vi "02señalizacion 492.vi"(5 "Digitales":T1, 6 "Analogicas":dbl[](array[numeric]), 7 "Config Equipo":T3={"Modelo"="", "IP"="", "Puerto"=0, "Time Out"=0, "Med Princ"=0, "Time sin rx"=60, "Reintento"=60, "Ref PD 2"=200} {"Ref PD 2" max=10000 step=1; "Med Princ" items=["1", "2", "3", "4", "5", "6", "7", "8", "9", "10", "11", "12", "13", "14", "15", "16", "17", "18", "19", "20", "21", "22", "23", "24", "25", "26", "27", "28", "29", "30", "31", "32"]}) -> (2 "Error Logico":bool, 3 "Señalizacion":T2)   [LabVIEW 2010]
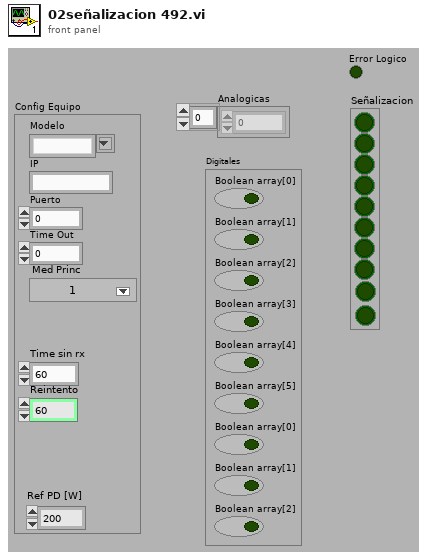
[diagram p1: front panel]
types:
  T1 = cluster{"Boolean array[0]":bool, "Boolean array[1]":bool, "Boolean array[2]":bool, "Boolean array[3]":bool, "Boolean array[4]":bool, "Boolean array[5]":bool, "Boolean array[0]":bool, "Boolean array[1]":bool, "Boolean array[2]":bool}
  T2 = cluster{bool, bool, bool, bool, bool, bool, bool, bool, bool, bool}
  T3 = cluster{"Modelo":string, "IP":string, "Puerto":u16, "Time Out":u16, "Med Princ":u16, "Time sin rx":u16, "Reintento":u16, "Ref PD 2":u16}
  T4 = cluster{bool, bool, bool, bool, bool, bool, bool, bool, bool, "Boolean array[5]":bool}
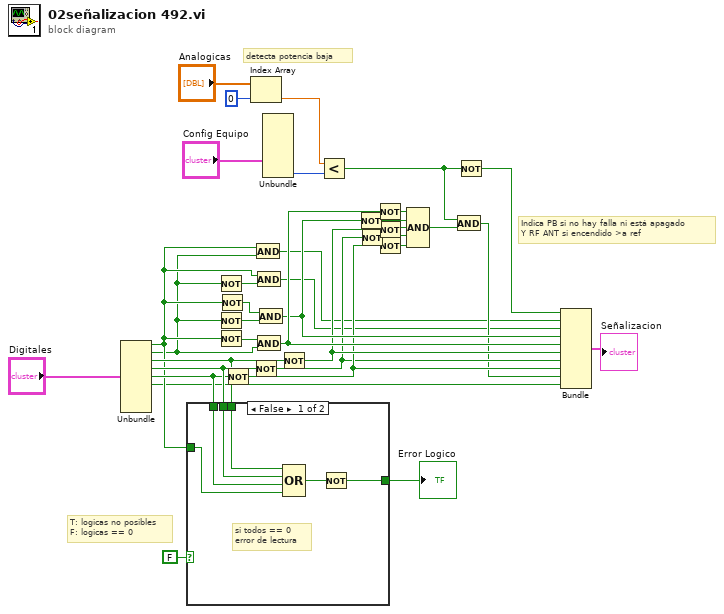
[diagram p0: block diagram]
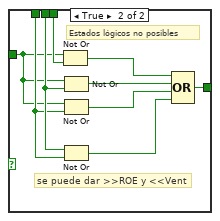
[diagram p2: hidden frame]
diagram:
  # "T: logicas no posibles\nF: logicas == 0"
  # "Indica PB si no hay falla ni está apagado\nY RF ANT si encendido >a ref"
  # "detecta potencia baja"
  n1 = Unbundle("Digitales") -> ("Boolean array[0]"=w29:bool, "Boolean array[1]"=w9:bool, "Boolean array[2]"=w31:bool, "Boolean array[3]"=w32:bool, "Boolean array[4]"=w30:bool, "Boolean array[5]"=w8:bool)  [unwired: 3 out]
  n2 = case shown="False" FALSE {
    tunnel: w32 -> [w40 w47]
    tunnel: w31 -> [w41 w46]
    tunnel: w30 -> [w39 w45]
    tunnel: w29 -> [w38 w44]
    tunnel: [w36 w43] -> w28
    frame False {
      # "si todos == 0\nerror de lectura"
      n3 = Compound Arithmetic op=OR(w41, w40, w39, w38) -> (w37:bool)
      n4 = Not(x=w37) -> (.not. x?=w36:bool)
    }
    frame True {
      # "se puede dar >>ROE y <<Vent"
      # "Estados lógicos no posibles"
      n5 = Not Or(1:w46, 2:w44) -> (0:w48:bool)
      n6 = Not Or(1:w47, 2:w44) -> (0:w49:bool)
      n7 = Not Or(1:w45, 2:w44) -> (0:w42:bool)
      n8 = Not Or(1:w45, 2:w47) -> (0:w50:bool)
      n9 = Compound Arithmetic op=OR(w48, w49, w42, w50) -> (w43:bool)
    }
  }
  "Error Logico" <- w28
  n10 = Not(x=w9) -> (.not. x?=w6:bool)
  n11 = Not(x=w9) -> (.not. x?=w5:bool)
  n12 = Not(x=w29) -> (.not. x?=w7:bool)
  n13 = Not(x=w29) -> (.not. x?=w4:bool)
  n14 = Not(x=w30) -> (.not. x?=w19:bool)
  n15 = Index Array(array="Analogicas", index=0 ("offset (0)")) -> (element=w27:dbl)
  n16 = Not(x=w32) -> (.not. x?=w18:bool)
  n17 = And(x=w29, y=w9) -> (x .and. y?=w12:bool)
  n18 = And(x=w29, y=w6) -> (x .and. y?=w13:bool)
  n19 = And(x=w7, y=w9) -> (x .and. y?=w24:bool)
  n20 = And(x=w4, y=w5) -> (x .and. y?=w23:bool)
  n21 = Unbundle("Config Equipo") -> ("Ref PD 2"=w33:u16)  [unwired: 7 out]
  n22 = Not(x=w31) -> (.not. x?=w20:bool)
  n23 = Less?(x=w27, y=w33) -> (x < y?=w2:bool)
  n24 = Not(x=w23) -> (.not. x?=w11:bool)
  n25 = Not(x=w18) -> (.not. x?=w21:bool)
  n26 = Not(x=w24) -> (.not. x?=w10:bool)
  n27 = Not(x=w20) -> (.not. x?=w22:bool)
  n28 = Not(x=w19) -> (.not. x?=w17:bool)
  n29 = Compound Arithmetic op=AND(w10, w11, w22, w21, w17) -> (w14:bool)
  n30 = And(x=w2, y=w14) -> (x .and. y?=w15:bool)
  n31 = Not(x=w2) -> (.not. x?=w1:bool)
  n32 = Bundle(w1, w12, w13, w23, w24, w20, w18, w19, w15, "Boolean array[5]"=w8) -> (→"Señalizacion":T4)  [unwired: 1 out]
